vi "BMonitor.vi"() -> ()   [LabVIEW 2016]
uses:
  Instrument_Setup.vi
  Global/Global Variables/Data_Display_global.vi
panel:
  out "String":string
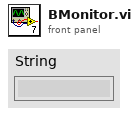
[diagram p1: front panel]
types:
  T1 = typedef "PSIO.ctl" = cluster{"Address":T2, "Version":enum16{"PS", "IPS"}}
  T2 = typedef "OxfordAddress.ctl" = cluster{"Com Port":i32, "ISOBUS Address":i32, "GPIB Address":i16, "Communication":enum16{"RS232", "ISOBUS", "GPIB", "Gateway"}}
  T3 = cluster{"Value":i16, "At rest":bool, "Sweeping":bool, "Rate limiting":bool}
  T4 = cluster{"Value":i16, "Hold":bool, "To set point":bool, "To zero":bool, "Clamped":bool}
  T5 = cluster{"Value":i16, "Off (at zero field)":bool, "On":bool, "Off (at field)":bool, "No switch fitted":bool, "Confirm":bool}
  T6 = cluster{"Value":i16, "Desired":u16, "Magnet":u16, "Commanded":u16, "Actual":u16}
  T7 = cluster{"Value":i16, "Quenched":bool, "Over heated":bool, "Warming up":bool}
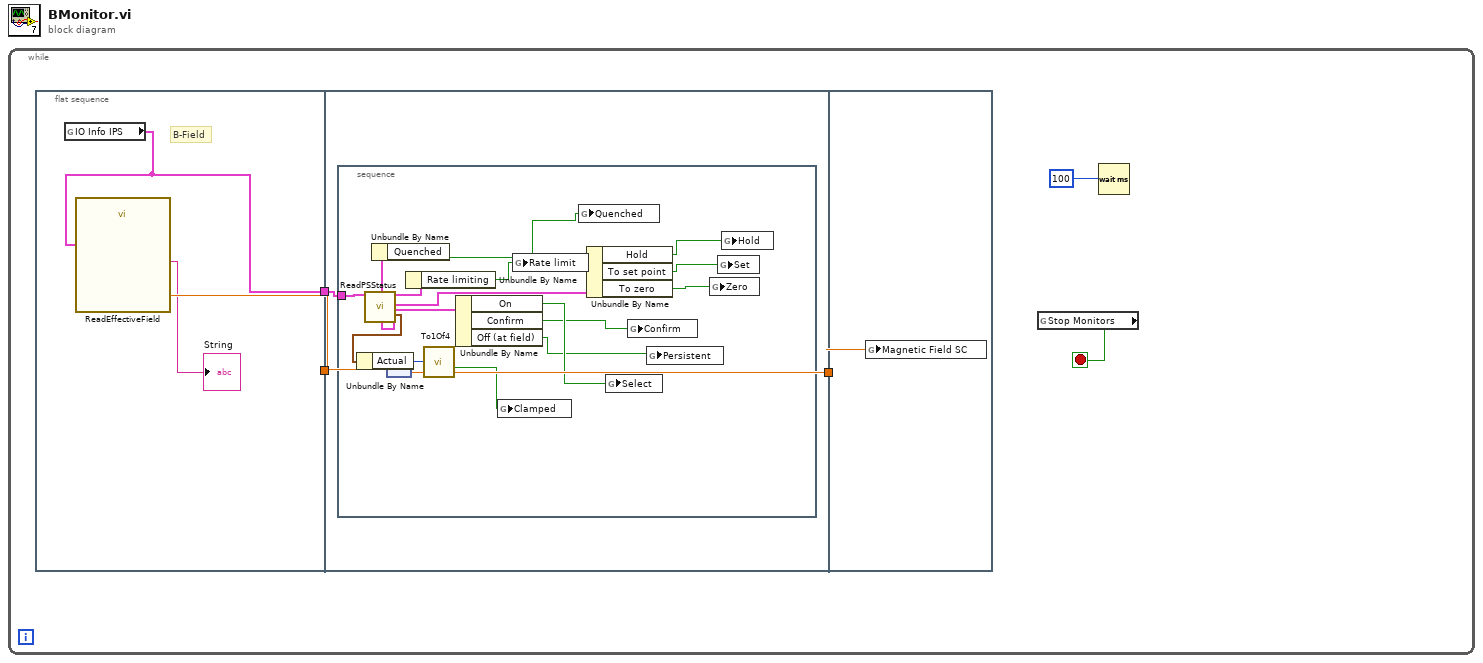
[diagram p0: block diagram]
diagram:
  n1 = while {
    stop <- w3 stop-if-true
    n2 = flat-sequence {
      tunnel: [w8] -> w5
      tunnel: [w6] -> w2
      tunnel: w5 -> [w11]
      tunnel: [w10] -> w4
      tunnel: w2 -> [w9]
      tunnel: w4 -> [w28]
      frame #0 {
        # "B-Field"
        n3 = global read "Instrument_Setup.vi" "IO Info IPS"() -> (w6:T1)
        n4 = call "ReadEffectiveField.vi"("IO Info"=w6) -> ("Effective field"=w8:dbl[unit], "Display"=→"String":string)  [unwired: 1 out]
      }
      frame #1 {
        n5 = stacked-sequence {
          tunnel: w9 -> [w26]
          frame #0 {
            n6 = call "ReadPSStatus.vi"("IO Info"=w26) -> ("Mode (n)"=w24:T3, "Activity"=w25:T4, "Switch Heater"=w23:T5, "Polarity"=w22:T6, "System Status (m)"=w21:T7)  [unwired: 10 in, 4 out]
            n7 = Unbundle By Name(w22) -> ("Actual"=w27:u16)
            n8 = Unbundle By Name(w21) -> ("Quenched"=w20:bool)
            n9 = Unbundle By Name(w24) -> ("Rate limiting"=w19:bool)
            n10 = call "To1Of4.vi"("Input"=w27) -> ("3"=w12:bool)  [unwired: 3 out]
            n11 = Unbundle By Name(w23) -> ("On"=w18:bool, "Confirm"=w16:bool, "Off (at field)"=w17:bool)
            n12 = global write "Data_Display_global.vi" "Clamped"(w12) -> ()
            n13 = global write "Data_Display_global.vi" "Rate limit"(w19) -> ()
            n14 = global write "Data_Display_global.vi" "Quenched"(w20) -> ()
            n15 = Unbundle By Name(w25) -> ("Hold"=w13:bool, "To set point"=w14:bool, "To zero"=w15:bool)
            n16 = global write "Data_Display_global.vi" "Select"(w18) -> ()
            n17 = global write "Data_Display_global.vi" "Confirm"(w16) -> ()
            n18 = global write "Data_Display_global.vi" "Persistent"(w17) -> ()
            n19 = global write "Data_Display_global.vi" "Zero"(w15) -> ()
            n20 = global write "Data_Display_global.vi" "Set"(w14) -> ()
            n21 = global write "Data_Display_global.vi" "Hold"(w13) -> ()
          }
        }
        n22 = node(w11) -> (w10:dbl)
      }
      frame #2 {
        n23 = global write "Data_Display_global.vi" "Magnetic Field SC"(w28) -> ()
      }
    }
    n24 = global read "Data_Display_global.vi" "Stop Monitors"() -> (w3:bool)
    n25 = Wait (ms)(milliseconds to wait=100) -> ()  [unwired: 1 out]
  }
